vi "ObtainQueue.vi"(8 "error in (no error)":errorcluster, 10 "create if not found? (f)":bool, 11 "ModuleAdmin":refnum<class "ModuleAdmin.lvclass">) -> (0 "error out":errorcluster, 2 "queue out":refnum<queue>, 3 "ModuleAdmin Out":refnum<class "ModuleAdmin.lvclass">)   [LabVIEW 2014, in "SpecAnModule.lvlib"]
doc: "This creates or recreates the queue name and obtains a reference to the queue."
uses:
  SpecAnModule.lvlib
  <userlib>/NIST/ModuleAdminLib/ModuleAdmin/ModuleAdmin.lvclass
  PublicAPI/Arguments/Messages/clMessage.ctl
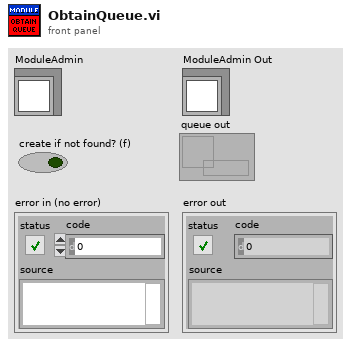
[diagram p1: front panel]
types:
  T1 = typedef "SpecAnModule.lvlib/clMessage.ctl" = cluster{"Message":string, "Message Data":variant}
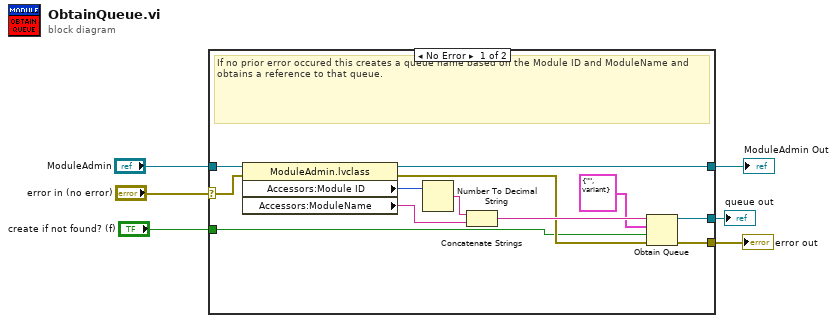
[diagram p0: block diagram]
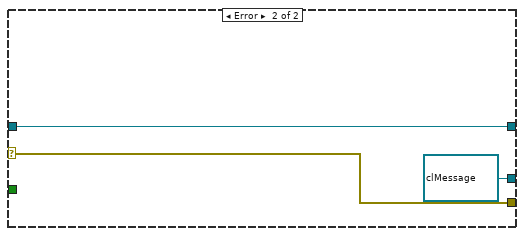
[diagram p2: hidden frame]
diagram:
  n1 = case shown="No Error" "error in (no error)" {
    selector: "error in (no error)" -> [w11 w21]
    tunnel: [w14 w21] -> w5
    tunnel: [w9 w20] -> w4
    tunnel: "ModuleAdmin" -> [w12 w20]
    tunnel: [w8 refnum<queue> refnum ("queue out")] -> w2
    tunnel: "create if not found? (f)" -> [w7 _]
    frame No Error {
      # "If no prior error occured this creates a queue name based on the Module ID and ModuleName and obtains a reference to that queue."
      n2 = property class="ModuleAdmin.lvclass"(reference=w12, error in=w11) -> (reference out=w9:refnum<class "ModuleAdmin.lvclass">, error out=w10:errorcluster, "Accessors:Module ID"=w17:i32, "Accessors:ModuleName"=w18:string)
      n3 = Number To Decimal String(number=w17) -> (decimal integer string=w15:string)  [unwired: 1 in]
      n4 = Concatenate Strings(w15, w18) -> (w16:string)
      n5 = Obtain Queue(name (unnamed)=w16, element data type=T1 {"Message"="", "Message Data"=variant} ("clMessage"), create if not found? (T)=w7, error in (no error)=w10) -> (queue out=w8:refnum<queue>, error out=w14:errorcluster)  [unwired: 1 in, 1 out]
    }
    frame Error {
    }
  }
  "error out" <- w5
  "ModuleAdmin Out" <- w4
  "queue out" <- w2
